vi "Shutdown Controller.vi"(5 "Purge Time":u32, 7 "Log File Refnum in":refnum<file>, 8 "error in":errorcluster, 9 "UI Data in":T2, 10 "Handshake Notifier in":refnum<notifier>, 11 "Message Queues in":T1) -> (0 "error out":errorcluster, 1 "UI Data out":T2, 2 "Handshake Notifier out":refnum<notifier>, 3 "Message Queues out":T1, 4 "Log File Refnum out":refnum<file>)   [LabVIEW 2014, in "Controller.lvlib"]
doc: "Shut down the boiler controller."
uses:
  Controller.lvlib
  controls/MHL UI Data.ctl
  controls/MHL Status.ctl
  support/Message Queue/All Message Queues.ctl
  support/Message Queue/Message Cluster.ctl
  support/Boiler System Globals.vi
  support/Message Queue/Message Queue.lvlib
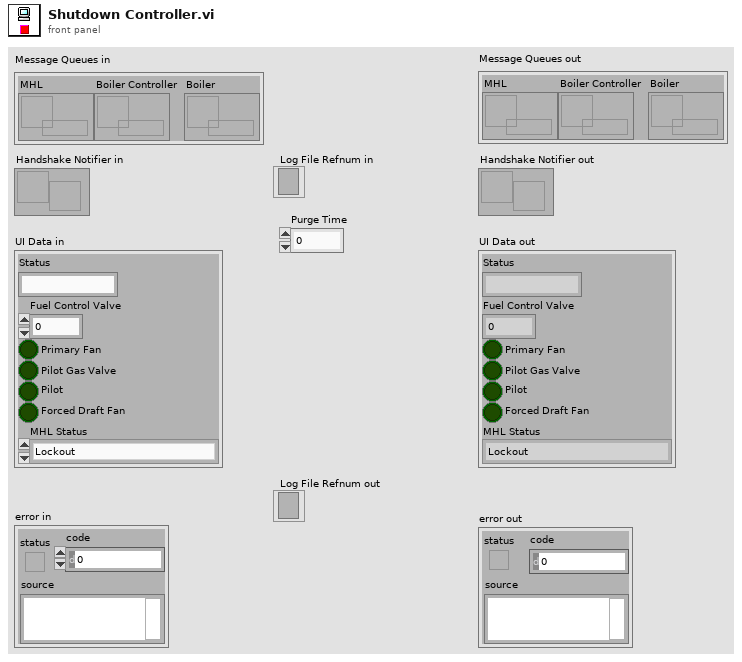
[diagram p1: front panel]
types:
  T1 = typedef "Message Queue.lvlib/All Message Queues.ctl" = cluster{"MHL":refnum<queue>, "Boiler Controller":refnum<queue>, "Boiler":refnum<queue>}
  T2 = typedef "MHL UI Data.ctl" = cluster{"Status":string, "Fuel Control Valve":u32, "Primary Fan":bool, "Pilot Gas Valve":bool, "Pilot":bool, "Forced Draft Fan":bool, "MHL Status":T3}
  T3 = typedef "MHL Status.ctl" = enum16{"Lockout", "Ready", "Pre-Purge", "Pre-Purge Complete", "Pilot On", "Boiler Running", "Shutdown", "Purge"}
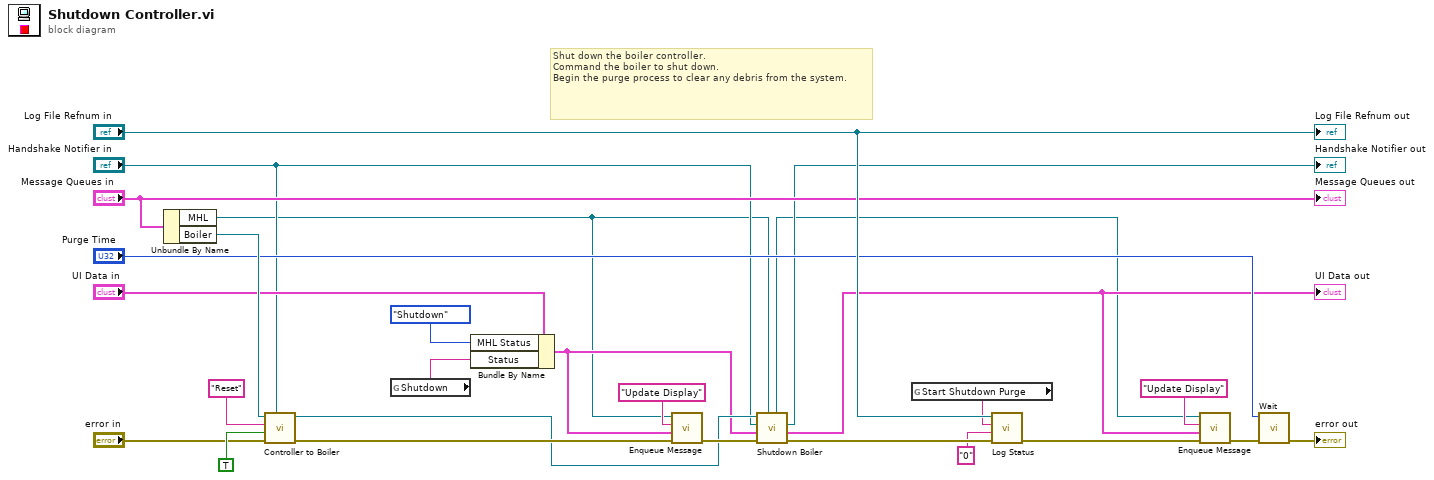
[diagram p0: block diagram]
diagram:
  # "Shut down the boiler controller. \nCommand the boiler to shut down.\nBegin the purge process to clear any debris from the system."
  n1 = Unbundle By Name("Message Queues in") -> ("MHL"=w2:refnum<queue>, "Boiler"=w16:refnum<queue>)
  n2 = call "Controller to Boiler.vi"("Notifier"="Handshake Notifier in", "error in"="error in", "Message Data"=TRUE ("Fuel Valve"), "Message"="Reset", "Boiler Queue in"=w16) -> ("error out"=w25:errorcluster, "Queue out"=w11:refnum<queue>)  [unwired: 4 in, 1 out]
  n3 = global read "Boiler System Globals.vi" "Shutdown"() -> (w10:string)
  n4 = Bundle By Name(cluster="UI Data in", "MHL Status"=MHL_Status."Shutdown", "Status"=w10) -> (w7:T2)
  n5 = call "Enqueue Message.vi"("error in (no error)"=w25, "Message Data"=w7, "Message"="Update Display", "Message Queue"=w2) -> ("error out"=w14:errorcluster)  [unwired: 6 in, 1 out]
  n6 = call "Shutdown Boiler.vi"("MHL Queue in"=w2, "error in"=w14, "UI Data in"=w7, "Handshake Notifier in"="Handshake Notifier in", "Boiler Queue in"=w11) -> ("error out"=w26:errorcluster, "UI Data out"=w6:T2, "Handshake Notifier out"=→"Handshake Notifier out":refnum<notifier>, "MHL Queue out"=w1:refnum<queue>)  [unwired: 2 in, 1 out]
  "UI Data out" <- w6
  n7 = global read "Boiler System Globals.vi" "Start Shutdown Purge"() -> (w9:string)
  n8 = call "Log Status.vi"("error in"=w26, "Event Data String (-)"="0" ("Event Data String"), "Event String"=w9, "Log File Refnum In"="Log File Refnum in") -> ("error out"=w18:errorcluster)  [unwired: 6 in, 1 out]
  n9 = call "Enqueue Message.vi"("error in (no error)"=w18, "Message Data"=w6, "Message"="Update Display", "Message Queue"=w1) -> ("error out"=w21:errorcluster)  [unwired: 6 in, 1 out]
  n10 = call "Wait.vi"("error in"=w21, "Purge Time (s)"="Purge Time") -> ("error out"=→"error out":errorcluster)  [unwired: 9 in]
  "Log File Refnum out" <- "Log File Refnum in"
  "Message Queues out" <- "Message Queues in"
